vi "host_open_form.vi"(8 "error in (no error)":errorcluster, 10 "JSON":string, 11 "name":string) -> (0 "error out":errorcluster)   [LabVIEW 2021]
uses:
  host_global_vars.vi
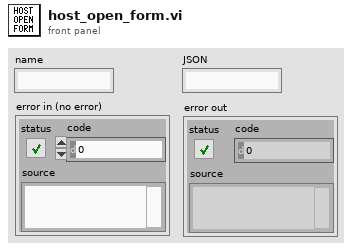
[diagram p1: front panel]
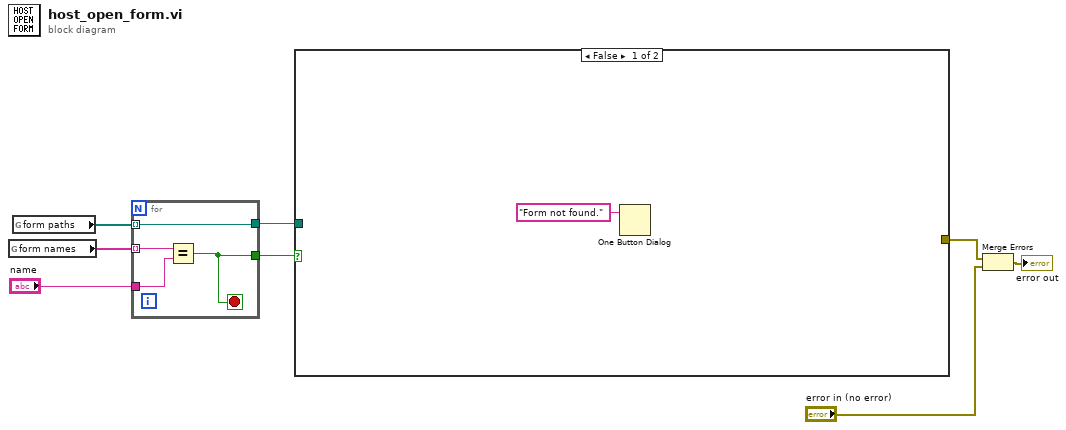
[diagram p0: block diagram]
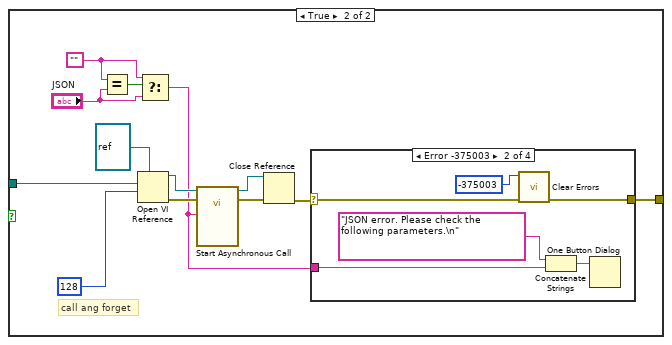
[diagram p2: hidden frame]
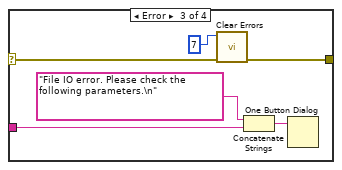
[diagram p4: hidden frame]
diagram:
  n1 = global read "host_global_vars.vi" "form names"() -> (w5:string[])
  n2 = global read "host_global_vars.vi" "form paths"() -> (w4:path[])
  n3 = for {
    tunnel: w5 -> [w12] mode=indexing
    tunnel: w4 -> [w10] mode=indexing
    tunnel: "name" -> [w11]
    tunnel: [w10] -> w2
    tunnel: [w9] -> w1
    stop <- w9 stop-if-true
    n4 = Equal?(x=w12, y=w11) -> (x = y?=w9:bool)
  }
  n5 = case shown="False" w1 {
    tunnel: [_ w16] -> w7
    tunnel: w2 -> [_ w14]
    frame False {
      n6 = One Button Dialog(message="Form not found.") -> ()  [unwired: 1 in, 1 out]
    }
    frame True {
      w18 = ""
      # "call ang forget"
      n7 = Equal?(x=w18, y="JSON") -> (x = y?=w19:bool)
      n8 = Open VI Reference(type specifier VI Refnum (for type only)=refnum<vi> refnum, vi path=w14, options=128) -> (vi reference=w23:refnum<vi>, error out=w24:errorcluster)  [unwired: 3 in]
      n9 = Select(t=w18, s=w19, f="JSON") -> (s? t:f=w15:string)
      n10 = call-by-ref "Start Asynchronous Call"(reference=w23, error in=w24, "JSON"=w15) -> (reference out=w21:refnum<vi>, error out=w22:errorcluster)  [unwired: 11 in]
      n11 = Close Reference(reference=w21, error in (no error)=w22) -> (error out=w20:errorcluster)
      n12 = case shown="Error -375003" w20 {
        selector: w20 -> [w27 w33 w39 w40]
        tunnel: [w27 w32 w38 w40] -> w16
        tunnel: w15 -> [_ w28 w34 _]
        frame No Error {
        }
        frame Error {
          n13 = call <vilib>:"Clear Errors.vi"("error in (no error)"=w33, "specific error code to clear (0: all)"=-375003) -> ("error out"=w32:errorcluster)  [unwired: 4 in, 1 out]
          n14 = Concatenate Strings("JSON error. Please check the following parameters.\n", w28) -> (w29:string)
          n15 = One Button Dialog(message=w29) -> ()  [unwired: 1 in, 1 out]
        }
        frame Error {
          n16 = call <vilib>:"Clear Errors.vi"("error in (no error)"=w39, "specific error code to clear (0: all)"=7) -> ("error out"=w38:errorcluster)  [unwired: 4 in, 1 out]
          n17 = Concatenate Strings("File IO error. Please check the following parameters.\n", w34) -> (w35:string)
          n18 = One Button Dialog(message=w35) -> ()  [unwired: 1 in, 1 out]
        }
        frame Default {
        }
      }
    }
  }
  n19 = Merge Errors(w7, "error in (no error)") -> (→"error out":errorcluster)
